vi "Do.vi"(8 "error in":errorcluster, 10 "Actor in":refnum<class "Actor.lvclass">, 11 "Write Device IDs Msg":refnum<class "Write Device IDs Msg.lvclass">) -> (0 "error out":errorcluster, 2 "Actor out":refnum<class "Actor.lvclass">)   [LabVIEW 2018, in "EMS User Interface Actor.lvlib" / "Write Device IDs Msg.lvclass"]
doc: "This VI delivers the message to the actor by calling the appropriate method(s) on the actor."
uses:
  Write Device IDs Msg.lvclass
  C:/Users/Administrator/Desktop/2018LabVIEW EMS/Dialog Actors/Devices to Load Actor/Devices to Load Messages/Return Devices to Load IDs Msg/Return Devices to Load IDs Msg.lvclass
  <vilib>/ActorFramework/Actor/Actor.lvclass
  EMS User Interface/EMS User Interface.lvclass
  C:/Program Files (x86)/National Instruments/LabVIEW 2018/vi.lib/ActorFramework/Actor/Actor.lvclass
  C:/Users/Administrator/Desktop/2018LabVIEW EMS/EMS Generic Actor/EMS Generic/EMS Generic.lvclass
  Dialog Actors/Devices to Load Actor/Devices to Load Messages/Return Devices to Load IDs Msg/Return Devices to Load IDs Msg.lvclass/Return Devices to Load IDs Msg.ctl
  EMS Generic Actor/EMS Generic/EMS Generic.lvclass
  Dialog Actors/Devices to Load Actor/Devices to Load Messages/Return Devices to Load IDs Msg/Return Devices to Load IDs Msg.lvclass
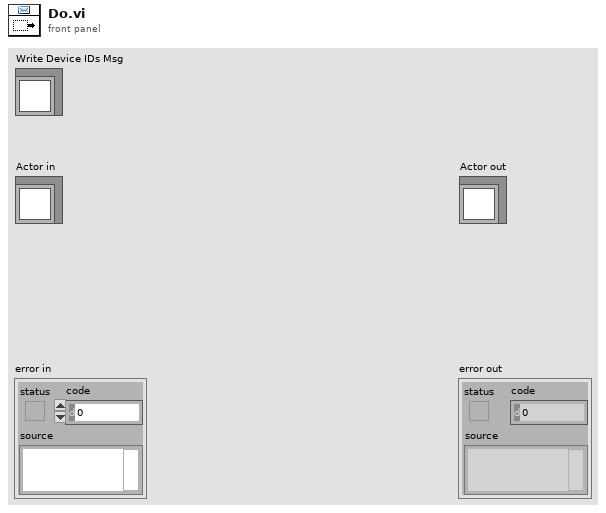
[diagram p1: front panel]
types:
  T1 = typedef "CSEISMIC DDS.lvlib/CSEISMIC DDS.lvclass/DeviceID.ctl" = string
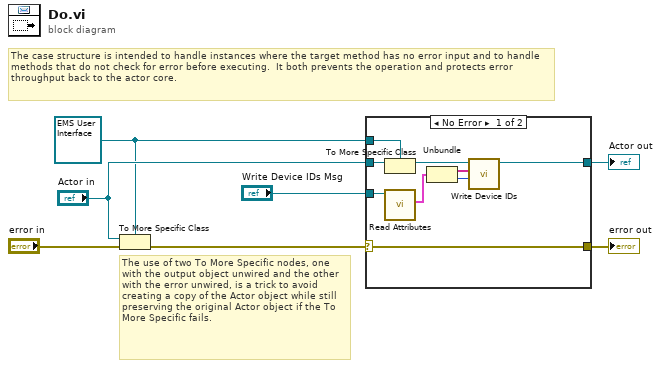
[diagram p0: block diagram]
diagram:
  w2 = refnum<class "EMS User Interface.lvclass"> refnum ("Actor in")
  # "The use of two To More Specific nodes, one with the output object unwired and the other with the error unwired, is a trick to avoid creating a copy of the Actor object while still preserving the original Actor object if the To More Specific fails."
  # "The case structure is intended to handle instances where the target method has no error input and to handle methods that do not check for error before executing.  It both prevents the operation and protects error throughput back to the actor core."
  n1 = To More Specific Class(target class=w2, reference="Actor in", error in="error in") -> (error out=w6:errorcluster)  [unwired: 1 out]
  n2 = case shown="No Error" w6 {
    selector: w6 -> [w15 w18]
    tunnel: [w15 w18] -> w5
    tunnel: [w16 w17] -> w4
    tunnel: "Actor in" -> [w14 w17]
    tunnel: w2 -> [w13 _]
    tunnel: "Write Device IDs Msg" -> [w10 _]
    frame No Error {
      n3 = To More Specific Class(target class=w13, reference=w14) -> (specific class reference=w12:refnum<class "EMS User Interface.lvclass">)  [unwired: 1 in, 1 out]
      n4 = call "Read Attributes.vi"("Return Devices to Load IDs Msg"=w10) -> ("Payload"=w11:cluster{"Device IDs":T1[], "Microgrid ID":u8})  [unwired: 10 in]
      n5 = Unbundle(w11) -> ("Device IDs"=w9:T1[], "Microgrid ID"=w8:u8)
      n6 = call "Write Device IDs.vi"("Microgrid ID"=w8, "Device ID Array"=w9, "EMS Generic in"=w12) -> ("dup EMS Generic out"=w16:refnum<class "EMS User Interface.lvclass">)  [unwired: 7 in, 1 out]
    }
    frame Error {
      # "If type check fails, pass the original object out again."
    }
  }
  "error out" <- w5
  "Actor out" <- w4
